vi "GDSAPI_CreateMethods.vi"(8 "error in (no error)":errorcluster, 10 "Methods":T3(array[cluster]), 11 "ClassPath(*.lvclass)":path) -> (0 "error out":errorcluster, 2 "MethodPath":path[](array[path]), 3 "ClassPathOut(*.lvclass)":path)   [LabVIEW 2014]
doc: "This VI creates Methods in a class."
uses:
  <resource>/Framework/Providers/Open_GDS/ClassProviders/Provider_EndevoGOOP300/GOOP300_SubVIs/GOOP300_MethodScopeType.ctl
  <resource>/Framework/Providers/Open_GDS/API/GDSAPI_SubVIs/GDSAPI_MethodType.ctl
  <resource>/Framework/Providers/Open_GDS/ClassProviders/Provider_BaseClassInterface/CreateMethodData.ctl
  <resource>/Framework/Providers/Open_GDS/ClassProviders/Provider_LvNativeClass/ClassWriterNative_class/IconDetails.ctl
  <resource>/Framework/Providers/Open_GDS/ClassProviders/Provider_LvNativeClass/ClassWriterNative_class/IconSize.ctl
  <resource>/Framework/Providers/Open_GDS/ClassProviders/Provider_LvNativeClass/ClassWriterNative_class/ClassWriterNative.lvclass
  <resource>/Framework/Providers/Open_GDS/ClassProviders/Provider_BaseClassInterface/ClassWriter_class/ClassWriter.lvclass
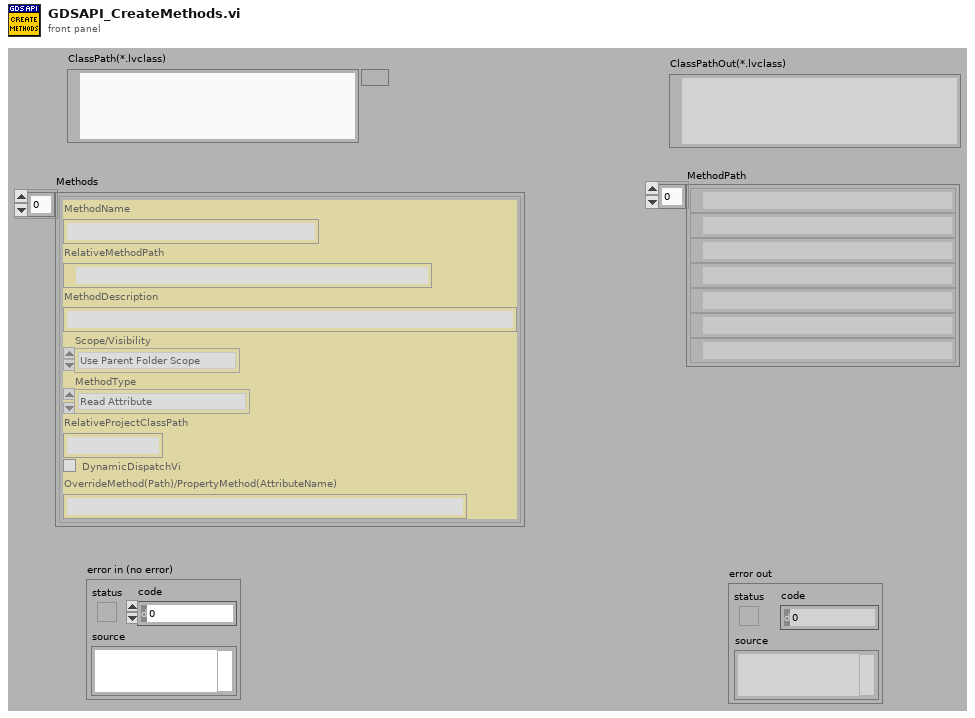
[diagram p1: front panel]
types:
  T1 = typedef "GOOP300_MethodScopeType.ctl" = enum16{"Use Parent Folder Scope", "Public", "Protected", "Private", "Community"}
  T2 = typedef "GDSAPI_MethodType.ctl" = enum16{"Read Attribute", "Write Attribute", "Read & Write Attribute", "None Modifying Method", "Get Property", "Set Property", "Read Property", "Write Property", "Static Method", "Interface Method"}
  T3 = cluster{"MethodName":string, "RelativeMethodPath":path, "MethodDescription":string, "Scope/Visibility":T1, "MethodType":T2, "RelativeProjectClassPath":string, "DynamicDispatchVi":bool, "OverrideMethod(Path)/PropertyMethod(AttributeName)":string}[]
  T4 = typedef "ClassWriter.lvclass/CreateMethodData.ctl" = cluster{"MethodName":string, "RelativeMethodPath":path, "MethodDescription":string, "Scope/Visibility":T1, "MethodTemplateName":string, "IconOut":u8[][], "RelativeProjectClassPath":string, "OpenViAfterCreation":bool, "DynamicDispatchVi":bool, "ExtraCreateParameters":variant, "MustOverride":bool, "MustCallParent":bool, "IconDetails":T5, "AF-Option":variant, "TemplatePath":path}
  T5 = typedef "ClassWriterNative.lvclass/IconDetails.ctl" = cluster{"IconSize":T6, "ImageRows(32)":i32, "ConnectorPaneHeight":i32[]}
  T6 = typedef "ClassWriterNative.lvclass/IconSize.ctl" = enum16{"Full", "1 c-term high", "2 c-term high", "3 c-term high"}
  T7 = cluster{"AttributeNames":string[], "PropertyNode":bool, "FolderNames":string[]}
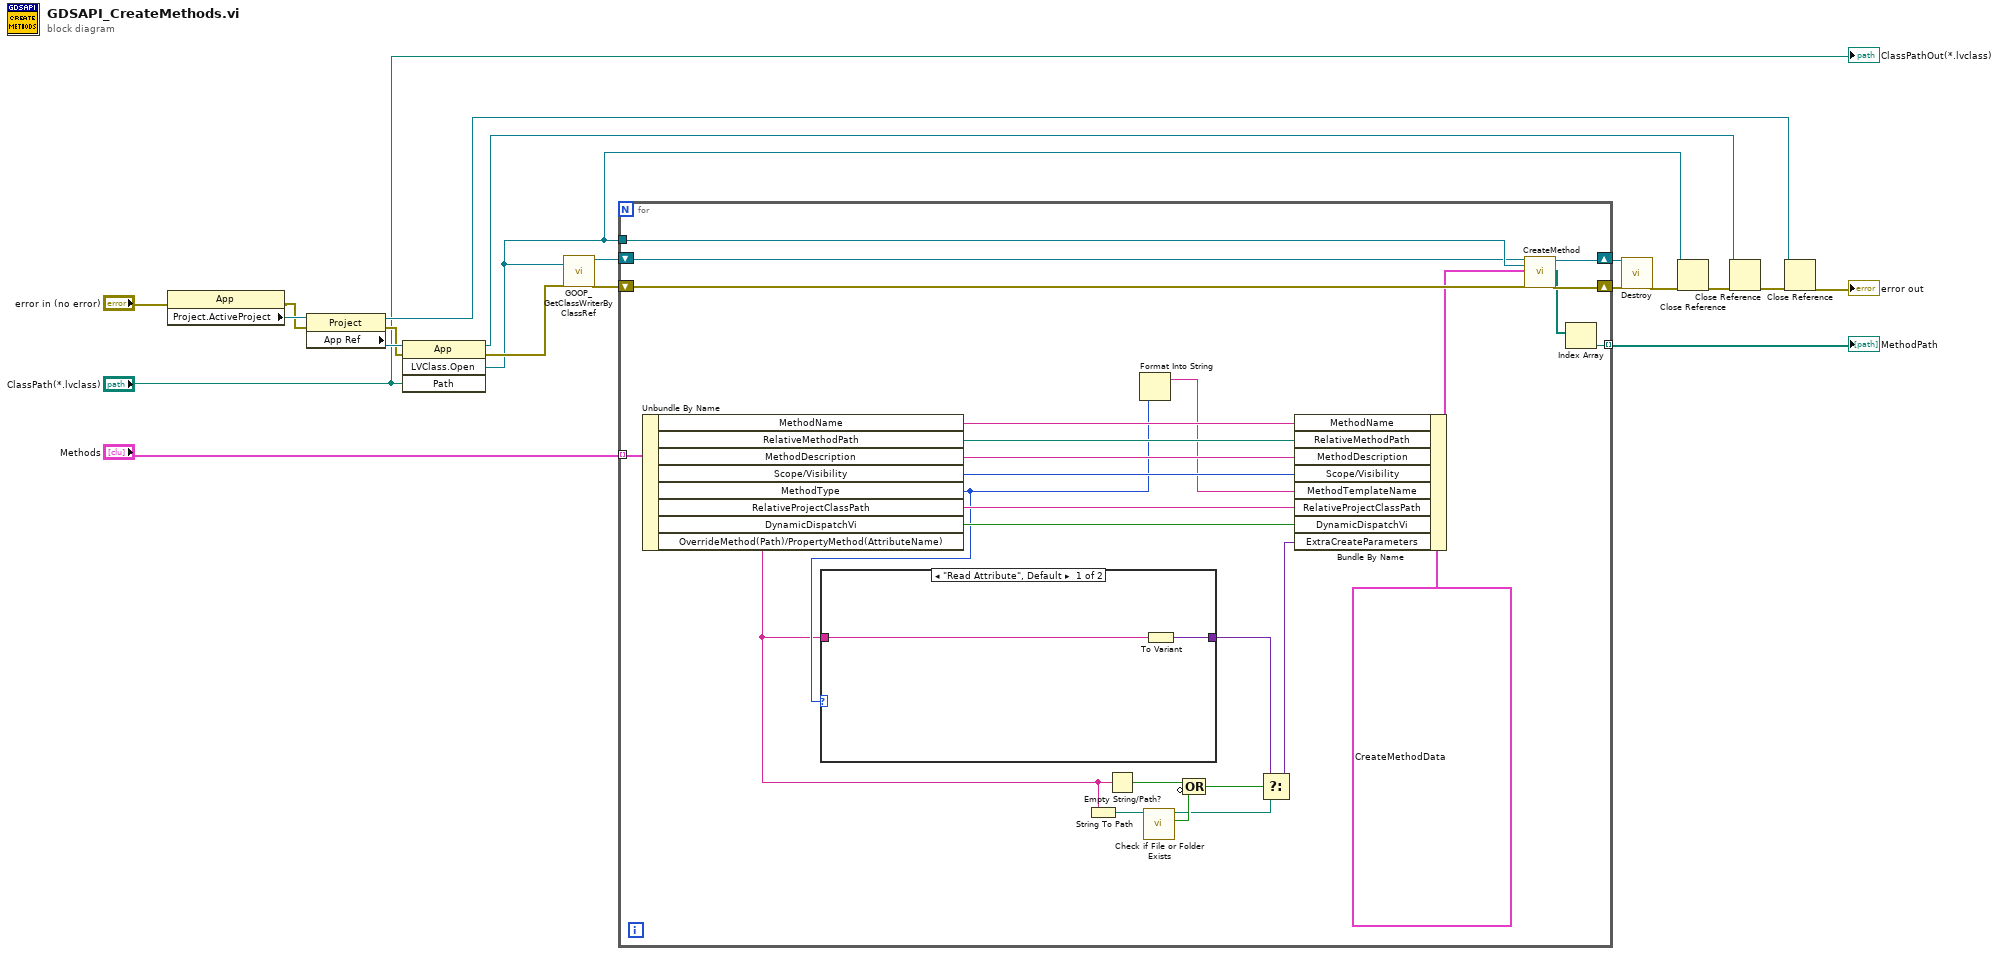
[diagram p0: block diagram]
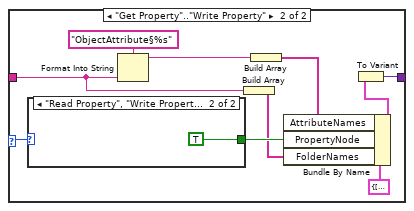
[diagram p2: hidden frame]
diagram:
  n1 = property class="App"(error in="error in (no error)") -> (error out=w9:errorcluster, "Project.ActiveProject"=w12:refnum<vi>)  [unwired: 1 in, 1 out]
  n2 = property class="Project"(reference=w12, error in=w9) -> (reference out=w4:refnum<vi>, error out=w10:errorcluster, "App Ref"=w11:refnum<vi>)
  n3 = invoke class="App" method="LVClass.Open"(reference=w11, error in=w10, "Path"="ClassPath(*.lvclass)") -> (reference out=w6:refnum<vi>, error out=w18:errorcluster, "LVClass.Open"=w13:refnum<vi>)  [unwired: 1 in, 1 out]
  n4 = call <resource>:"GOOP_GetClassWriterByClassRef.vi"("LVClassLibrary Refnum"=w13, "error in (no error)"=w18) -> ("ClassWriterNative.lvclass"=w14:refnum<class "ClassWriterNative.lvclass">, "error out"=w15:errorcluster)  [unwired: 16 in]
  n5 = for {
    tunnel: w13 -> [w43]
    tunnel: "Methods" -> [w27] mode=indexing
    shift-right: [w45] -> w16
    shift-left: w15 -> [w44]
    shift-right: [w46] -> w17
    shift-left: w14 -> [w42]
    tunnel: [w21] -> w1 mode=indexing
    n6 = Unbundle By Name(w27) -> ("MethodName"=w40:string, "RelativeMethodPath"=w39:path, "MethodDescription"=w38:string, "Scope/Visibility"=w37:T1, "MethodType"=w25:T2, "RelativeProjectClassPath"=w36:string, "DynamicDispatchVi"=w35:bool, "OverrideMethod(Path)/PropertyMethod(AttributeName)"=w24:string)
    n7 = case shown="\"Read Attribute\", Default" w25 {
      selector: w25 -> [_ w56]
      tunnel: w24 -> [w48 w52]
      tunnel: [w47 w49] -> w23
      frame "Read Attribute", Default {
        n8 = To Variant(anything=w48) -> (Variant=w47:variant)
      }
      frame "Get Property".."Write Property" {
        n9 = case shown="\"Read Property\", \"Write Property\"" w56 {
          tunnel: [_ TRUE ("PropertyNode")] -> w57
          frame "Read Attribute", Default {
          }
          frame "Read Property", "Write Property" {
          }
        }
        n10 = Format Into String(format string="ObjectAttribute§%s", w52) -> (resulting string=w54:string)  [unwired: 2 in, 1 out]
        n11 = Build Array(w52) -> (w51:string[])
        n12 = Build Array(w54) -> (w53:string[])
        n13 = Bundle By Name(cluster=T7 {"AttributeNames"=[], "PropertyNode"=FALSE, "FolderNames"=[]}, "AttributeNames"=w53, "PropertyNode"=w57, "FolderNames"=w51) -> (w50:T7)
        n14 = To Variant(anything=w50) -> (Variant=w49:variant)
      }
    }
    n15 = String To Path(string=w24) -> (path=w34:path)
    n16 = Empty String/Path?(string/path=w24) -> (empty?=w32:bool)
    n17 = Format Into String(w25) -> (resulting string=w26:string)  [unwired: 3 in, 1 out]
    n18 = call <vilib>:"Check if File or Folder Exists.vi"("path"=w34) -> ("file or folder exists?"=w33:bool, "dup path"=w30:path)  [unwired: 8 in, 1 out]
    n19 = Compound Arithmetic op=OR(w32, invert w33) -> (w31:bool)
    n20 = Select(t=w23, s=w31, f=w30) -> (s? t:f=w29:variant)
    n21 = Bundle By Name(cluster=T4 {"MethodName"="", "RelativeMethodPath"=path "", "MethodDescription"="", "Scope/Visibility"=enum."Use Parent Folder Scope", "MethodTemplateName"="", "IconOut"=[], "RelativeProjectClassPath"="", "OpenViAfterCreation"=FALSE, "DynamicDispatchVi"=FALSE, "ExtraCreateParameters"=variant, "MustOverride"=FALSE, "MustCallParent"=FALSE, "IconDetails"={"IconSize"=enum."Full", "ImageRows(32)"=0, "ConnectorPaneHeight"=[]}, "AF-Option"=variant, "TemplatePath"=path ""} ("CreateMethodData"), "MethodName"=w40, "RelativeMethodPath"=w39, "MethodDescription"=w38, "Scope/Visibility"=w37, "MethodTemplateName"=w26, "RelativeProjectClassPath"=w36, "DynamicDispatchVi"=w35, "ExtraCreateParameters"=w29) -> (w28:T4)
    n22 = call-dynamic "CreateMethod.vi"("ClassWriterNative.lvclass"=w42, "ClassItemRefIn"=w43, "CreateMethodData"=w28, "error in (no error)"=w44) -> ("ClassWriterNative.lvclass 2"=w46:refnum<class "ClassWriterNative.lvclass">, "MethodPaths"=w22:path[], "error out"=w45:errorcluster)  [unwired: 12 in, 1 out]
    n23 = Index Array(array=w22) -> (element=w21:path)  [unwired: 1 in]
  }
  "MethodPath" <- w1
  n24 = call-dynamic "Destroy.vi"("ClassWriterNative"=w17, "error in (no error)"=w16) -> ("error out"=w19:errorcluster)  [unwired: 17 in]
  n25 = Close Reference(reference=w13, error in (no error)=w19) -> (error out=w7:errorcluster)
  n26 = Close Reference(reference=w6, error in (no error)=w7) -> (error out=w5:errorcluster)
  n27 = Close Reference(reference=w4, error in (no error)=w5) -> (error out=→"error out":errorcluster)
  "ClassPathOut(*.lvclass)" <- "ClassPath(*.lvclass)"
